vi "output_create-open.vi"() -> ()   [LabVIEW 2016]
panel:
  in  "error in":errorcluster
  out "error out":errorcluster
  out "refnum out":refnum<file>
  out "Output File Path":path
  out "Output File Name":string
  in  "Output Folder Path":path
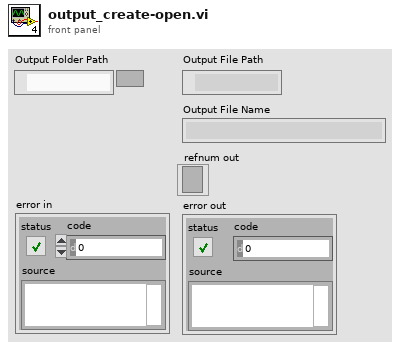
[diagram p1: front panel]
types:
  T1 = enum16{"open", "replace", "create", "open or create", "replace or create", "replace or create with confirmation"}
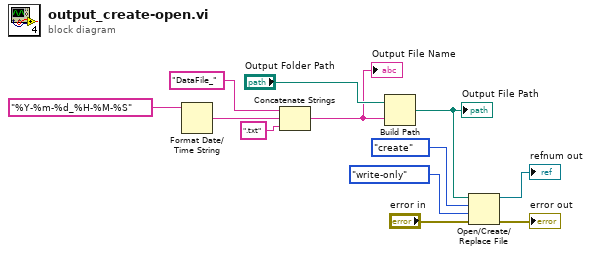
[diagram p0: block diagram]
diagram:
  n1 = Format Date/Time String(time format string (%c)="%Y-%m-%d_%H-%M-%S") -> (date/time string=w8:string)  [unwired: 2 in]
  n2 = Concatenate Strings("DataFile_" ("string"), w8, ".txt" ("string")) -> (w1:string)
  "Output File Name" <- w1
  n3 = Build Path(base path="Output Folder Path", name or relative path=w1) -> (appended path=w5:path)
  "Output File Path" <- w5
  n4 = Open/Create/Replace File(file path (use dialog)=w5, error in="error in", operation (0:open)=T1."create", access (0:read/write)=enum16{"read/write", "read-only", "write-only"}."write-only") -> (refnum out=→"refnum out":refnum<file>, error out=→"error out":errorcluster)  [unwired: 2 in, 1 out]
